vi "wsRegisteredEvents.vi"(9 "msgID":string, 10 "Event Name (empty =all)":string, 11 "Action":T1) -> (0 "Event Name":string, 1 "Found?":bool, 2 "Found ID":string, 3 "Array":T2[](array[typedef]))   [LabVIEW 2018, in "HASS-LV-WS_integration.lvlib"]
uses:
  HASS-LV-WS_integration.lvlib
  TypeDef/eventIDlistTypeDef.ctl
  TypeDef/registeredEventTypeDef.ctl
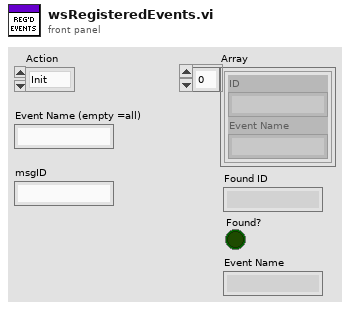
[diagram p1: front panel]
types:
  T1 = typedef "HASS-LV-WS_integration.lvlib/registeredEventTypeDef.ctl" = enum16{"Init", "Register", "Unregister", "Get MSG ID", "Get Event Name", "Get All Events"}
  T2 = typedef "HASS-LV-WS_integration.lvlib/eventIDlistTypeDef.ctl" = cluster{"ID":string, "Event Name":string}
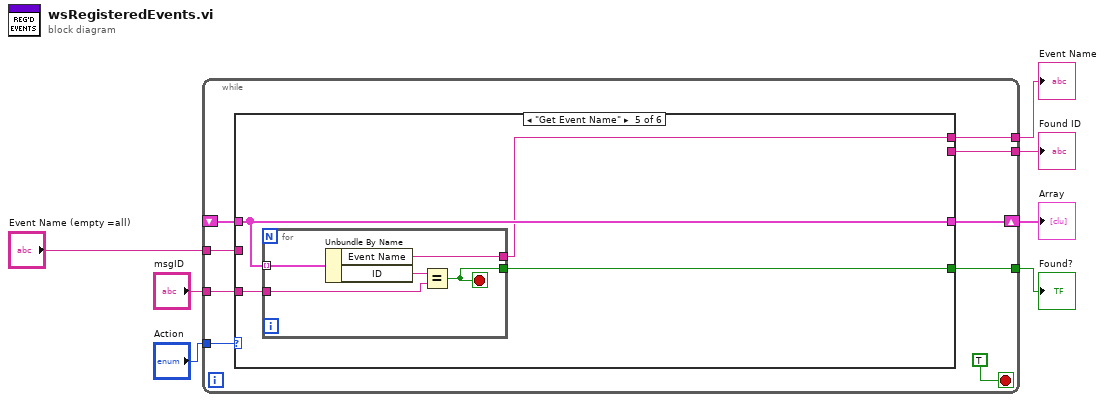
[diagram p0: block diagram]
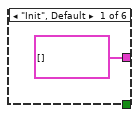
[diagram p2: hidden frame]
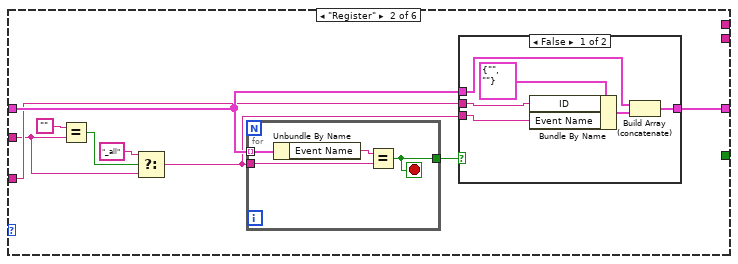
[diagram p3: hidden frame]
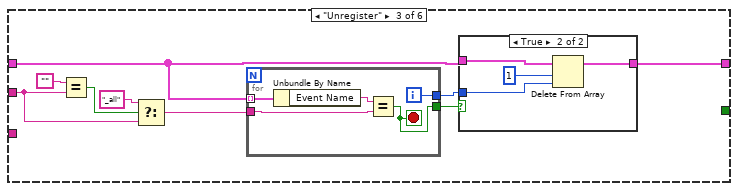
[diagram p5: hidden frame]
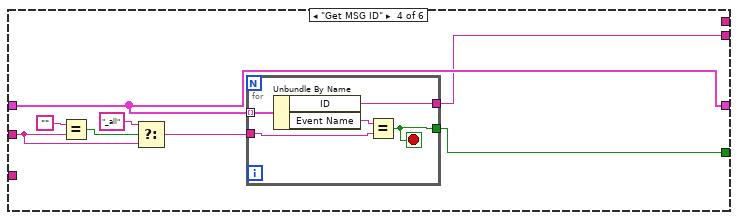
[diagram p7: hidden frame]
diagram:
  n1 = while {
    tunnel: "Action" -> [w15]
    shift-right: [w14] -> w7
    shift-left: _ -> [w13]
    tunnel: "Event Name (empty =all)" -> [w12]
    tunnel: "msgID" -> [w11]
    tunnel: [w10] -> w3
    tunnel: [w9] -> w2
    tunnel: [w8] -> w1
    stop <- TRUE stop-if-true
    n2 = case shown="\"Get Event Name\"" w15 {
      tunnel: [T2[] [] w24 w39 w64 w72 w79] -> w14
      tunnel: w13 -> [_ w25 w40 w64 w72 w79]
      tunnel: w12 -> [_ w20 w43 w58 _ _]
      tunnel: w11 -> [_ w23 _ _ w73 _]
      tunnel: [_ _ _ w63 _ _] -> w10
      tunnel: [_ _ _ w62 w71 _] -> w9
      tunnel: [_ _ _ _ w70 _] -> w8
      frame "Init", Default {
      }
      frame "Register" {
        n3 = Equal?(x="", y=w20) -> (x = y?=w21:bool)
        n4 = Select(t="_all", s=w21, f=w20) -> (s? t:f=w18:string)
        n5 = for {
          tunnel: w25 -> [w37] mode=indexing
          tunnel: w18 -> [w35]
          tunnel: [w34] -> w26
          stop <- w34 stop-if-true
          n6 = Unbundle By Name(w37) -> ("Event Name"=w36:string)
          n7 = Equal?(x=w36, y=w35) -> (x = y?=w34:bool)
        }
        n8 = case shown="False" w26 {
          tunnel: w25 -> [w32 w33]
          tunnel: [w31 w33] -> w24
          tunnel: w23 -> [w28 _]
          tunnel: w18 -> [w27 _]
          frame False {
            n9 = Bundle By Name(cluster=T2 {"ID"="", "Event Name"=""} ("Cluster"), "ID"=w28, "Event Name"=w27) -> (w29:T2)
            n10 = Build Array (concatenate)(w32, w29) -> (w31:T2[])
          }
          frame True {
          }
        }
      }
      frame "Unregister" {
        n11 = Equal?(x="", y=w43) -> (x = y?=w45:bool)
        n12 = Select(t="_all", s=w45, f=w43) -> (s? t:f=w42:string)
        n13 = for {
          tunnel: w40 -> [w56] mode=indexing
          tunnel: w42 -> [w54]
          tunnel: [w53] -> w41
          tunnel: [w52] -> w38
          i -> [w52]
          stop <- w53 stop-if-true
          n14 = Unbundle By Name(w56) -> ("Event Name"=w55:string)
          n15 = Equal?(x=w55, y=w54) -> (x = y?=w53:bool)
        }
        n16 = case shown="True" w41 {
          tunnel: w40 -> [w47 w51]
          tunnel: [w47 w50] -> w39
          tunnel: w38 -> [_ w48]
          frame False {
          }
          frame True {
            n17 = Delete From Array(array=w51, length=1, index=w48) -> (array with subset deleted=w50:T2[])  [unwired: 1 out]
          }
        }
      }
      frame "Get MSG ID" {
        n18 = Equal?(x="", y=w58) -> (x = y?=w60:bool)
        n19 = Select(t="_all", s=w60, f=w58) -> (s? t:f=w57:string)
        n20 = for {
          tunnel: w64 -> [w69] mode=indexing
          tunnel: w57 -> [w67]
          tunnel: [w66] -> w63
          tunnel: [w65] -> w62
          stop <- w65 stop-if-true
          n21 = Unbundle By Name(w69) -> ("ID"=w66:string, "Event Name"=w68:string)
          n22 = Equal?(x=w68, y=w67) -> (x = y?=w65:bool)
        }
      }
      frame "Get Event Name" {
        n23 = for {
          tunnel: w72 -> [w78] mode=indexing
          tunnel: w73 -> [w76]
          tunnel: [w75] -> w70
          tunnel: [w74] -> w71
          stop <- w74 stop-if-true
          n24 = Unbundle By Name(w78) -> ("Event Name"=w75:string, "ID"=w77:string)
          n25 = Equal?(x=w77, y=w76) -> (x = y?=w74:bool)
        }
      }
      frame "Get All Events" {
      }
    }
  }
  "Array" <- w7
  "Found ID" <- w3
  "Found?" <- w2
  "Event Name" <- w1
